vi "02_dosing.vi"() -> ()   [LabVIEW 2024]
uses:
  <vilib>/Utility/error.llb/DialogType.ctl
  <vilib>/Waveform/WDTOps.llb/WDT Waveform to XY Pairs DBL.vi
  <vilib>/Instr/_visa.llb/VISA Configure Serial Port (Instr).vi
  <vilib>/Utility/file.llb/Write Delimited Spreadsheet (string).vi
  <instrlib>/Tektronix DMM40x0 Series/Tektronix DMM40x0 Series.lvlib
panel:
  out "Waveform Graph":dbl[](graph)
  out "XY pairs":cluster{"x":timestamp, "y":dbl}[](array[cluster]) {"y" format="%0.2f"}
  in  "stop 2":bool
  in  "start   3":bool
  in  "pulse   2":bool
  in  "ready   2":bool
  in  "String 2":string
  out "String":string
  in  "Timeout (10000 ms)":u32=10000
  in  "Sample Count (10)":i32=10 format="%#.6g"
  in  "Trigger Count (5)":i32=5 format="%#.6g"
  in  "Function (0: DC Voltage)":u16(ring) items=["DC Voltage", "AC Voltage", "2 - Wire Resistance", "4 - Wire Resistance", "DC Current", "AC Current", "Frequency", "Period", "Continuity", "Diode Checking", "Temperature", "Capacitance"]
  in  "Serial Configuration":T1={"Baud Rate"=9600, "Parity"=0, "Data Bits"=8, "Stop Bits"=10, "Flow Control"=0} {"Flow Control" items=["None", "XON/XOFF", "RTS/CTS", "XON/XOFF & RTS/CTS", "DTR/DSR", "XON/XOFF & DTR/DSR"]; "Stop Bits" items=["1.0"=10, "1.5"=15, "2.0"=20]; "Data Bits" items=["7"=7, "8"=8]; "Parity" items=["None", "Odd", "Even", "Mark", "Space"]; "Baud Rate" items=["300"=300, "600"=600, "1200"=1200, "2400"=2400, "4800"=4800, "9600"=9600, "19200"=19200]}
  in  "VISA resource name":refnum<visa-resource-name>
  out "Data":string
  out "Array":string[](array[string])
  in  "SERIAL COMMAND":string(combo)
  out "PH METER OUTPUT":string
  in  "stop":bool
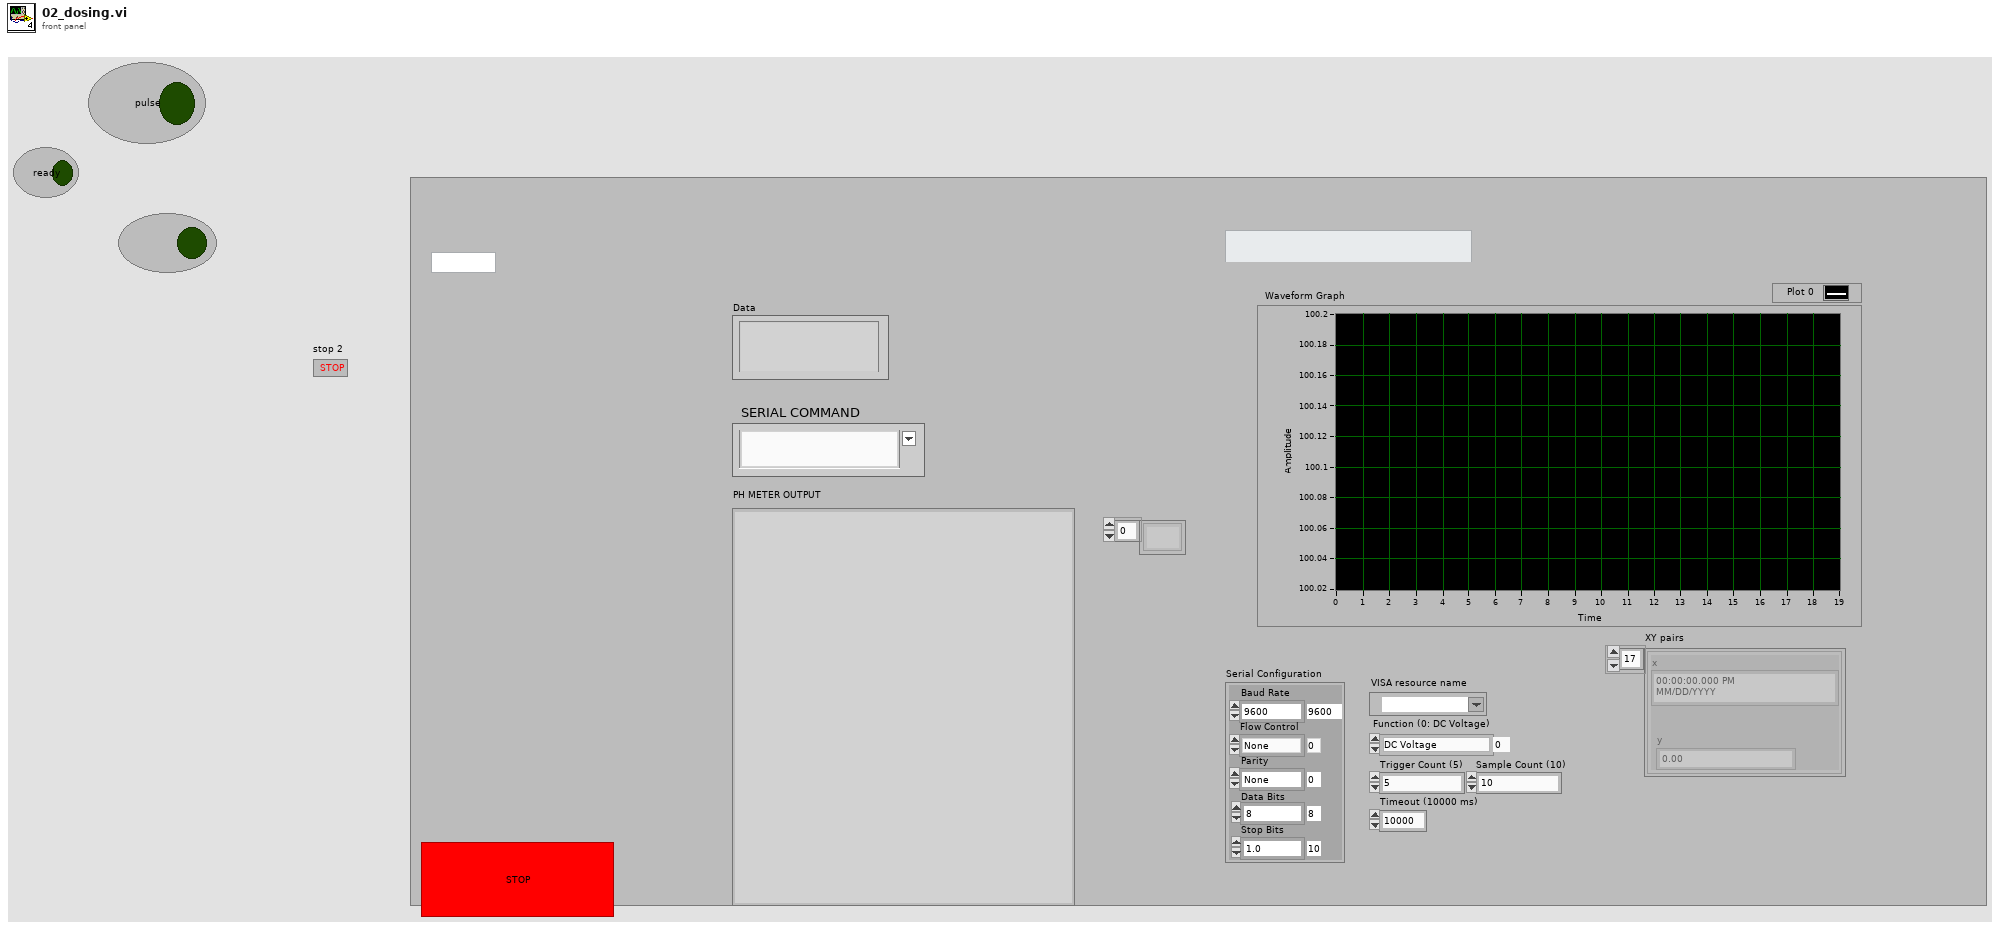
[diagram p1: front panel]
types:
  T1 = cluster{"Baud Rate":u32, "Parity":u16, "Data Bits":u16, "Stop Bits":u16, "Flow Control":u16}
  T2 = typedef "DialogType.ctl" = u16
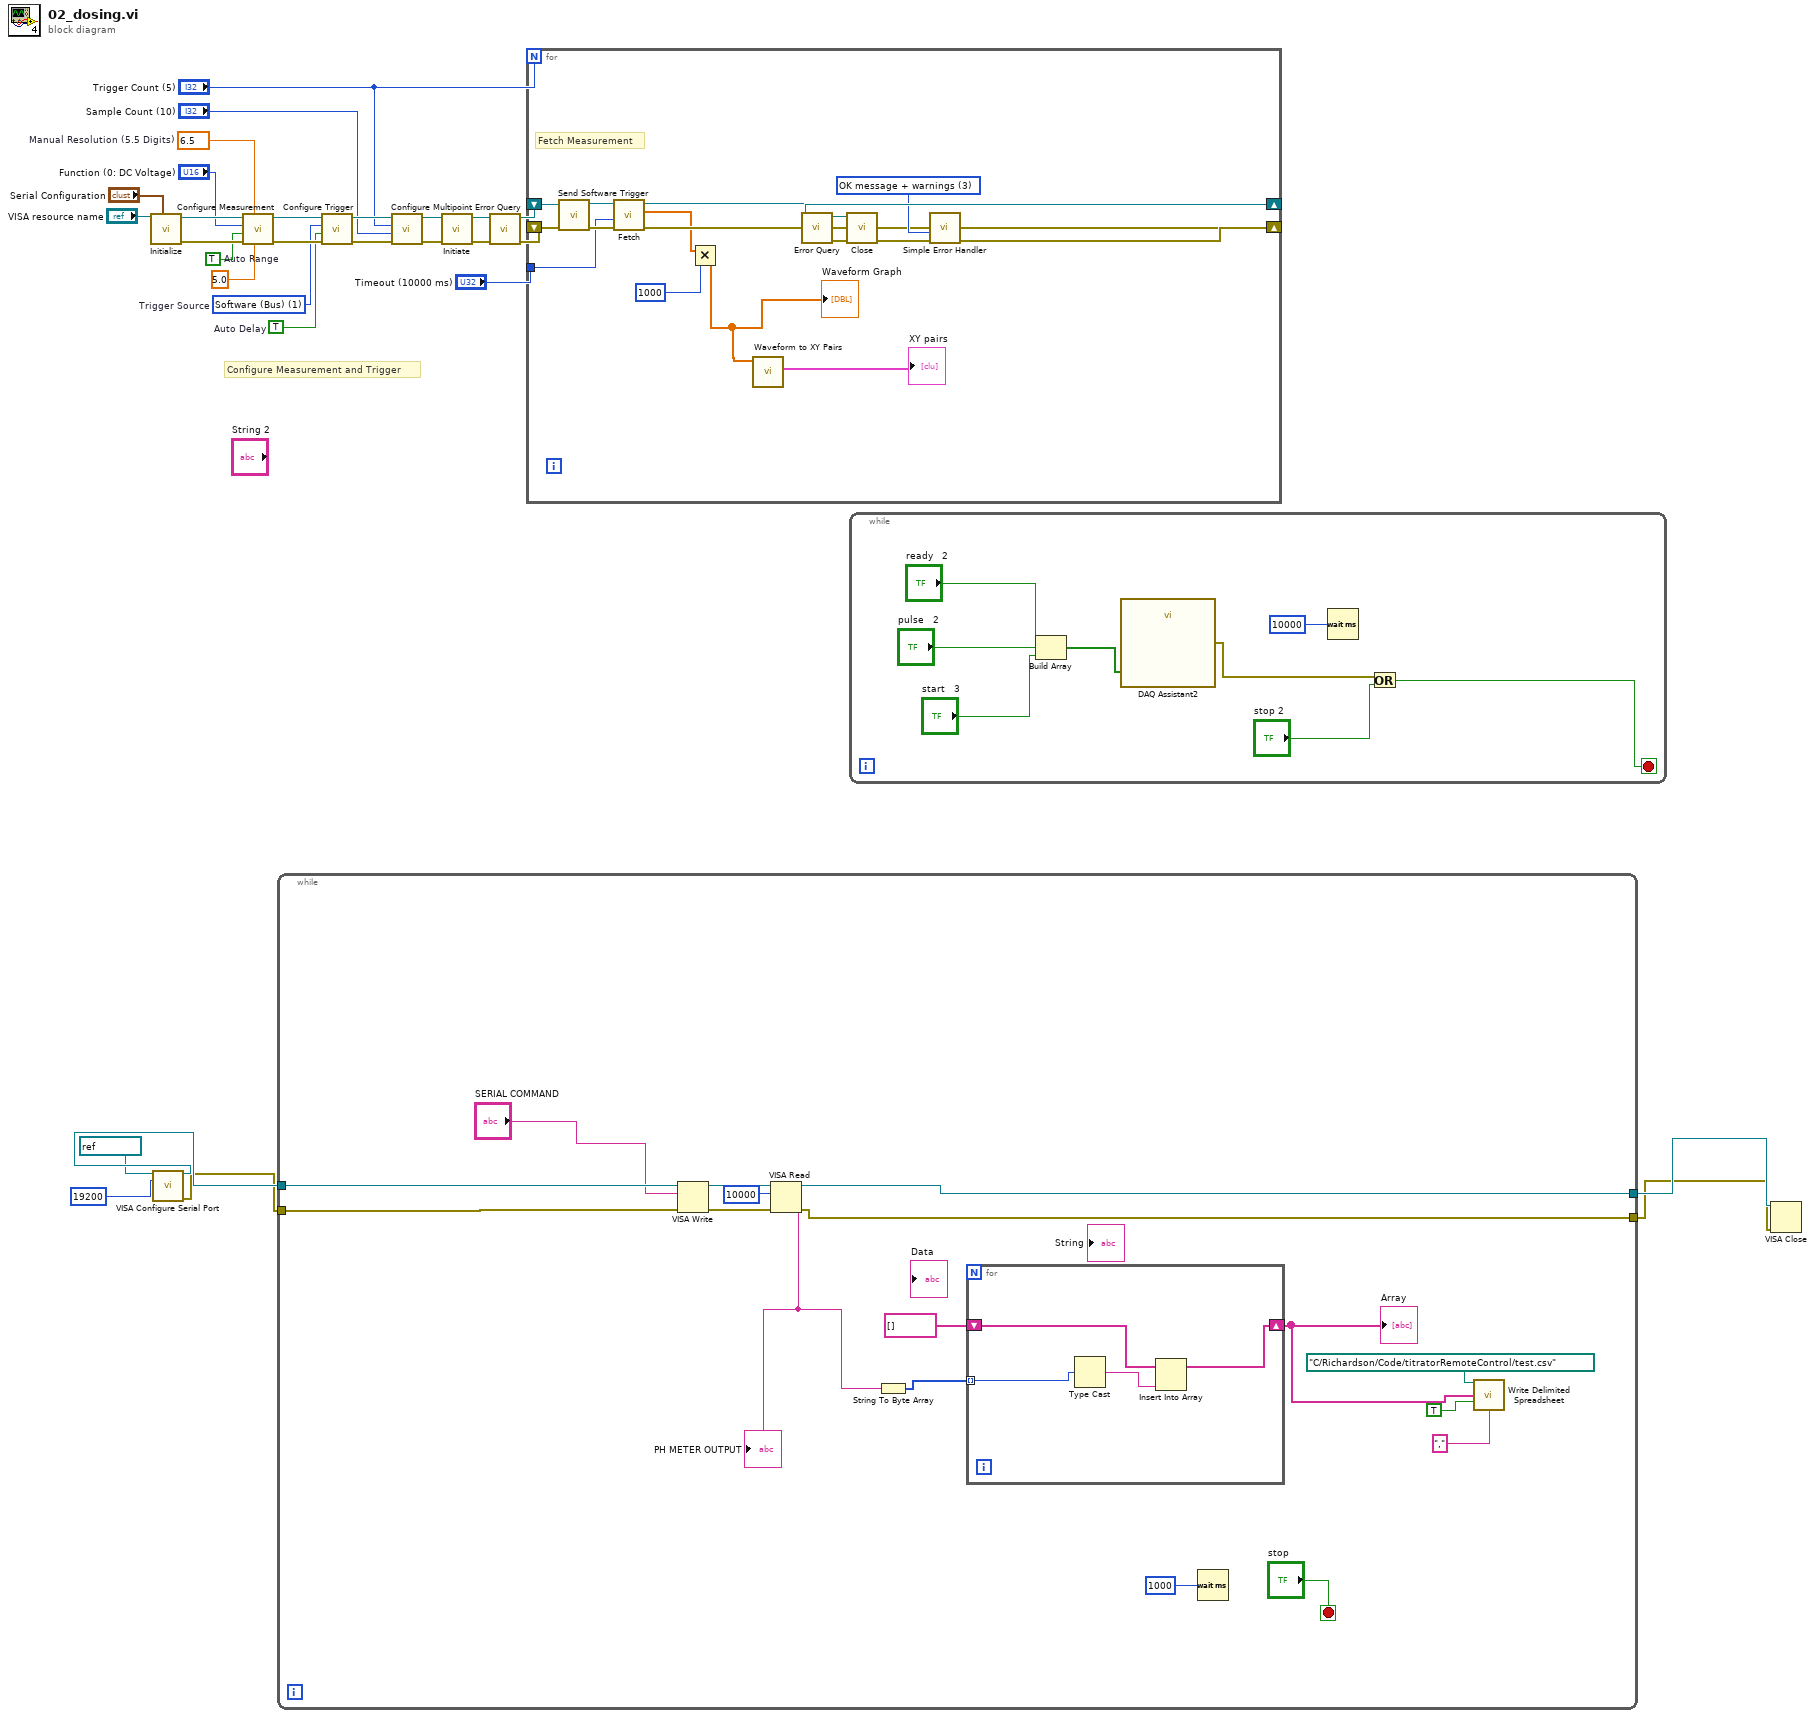
[diagram p0: block diagram]
diagram:
  w4 = 6.5 items=["4.5"=4.5, "5.5"=5.5, "6.5"=6.5]  # Manual Resolution (5.5 Digits)
  w12 = TRUE  # Auto Delay
  w13 = u16 1 items=["Immediate", "Software (Bus)", "External"]  # Trigger Source
  w14 = TRUE  # Auto Range
  w17 = T2 3 items=["no dialog", "OK message", "continue or stop message", "OK message + warnings", "continue/stop + warnings"] ("type of dialog (OK msg:1)")
  # "Configure Measurement and Trigger"
  n1 = call <instrlib>:"Initialize.vi"("Serial Configuration"="Serial Configuration", "VISA resource name"="VISA resource name") -> ("error out"=w29:errorcluster, "VISA resource name out"=w30:refnum<visa-resource-name>)  [unwired: 3 in, 5 out]
  n2 = call-poly "VISA Configure Serial Port"("VISA resource name"=refnum<visa-resource-name> "COM6", "baud rate (9600)"=u32 19200 ("byte count")) -> ("VISA resource name out"=w35:refnum<visa-resource-name>, "error out"=w33:errorcluster)  [unwired: 12 in]
  n3 = call <instrlib>:"Configure Measurement.vi"("Manual Range (1.0)"=5.0, "Manual Resolution (5.5 Digits)"=w4, "error in (no error)"=w29, "Auto Range (T:Enable)"=w14, "Function (0: DC Voltage)"="Function (0: DC Voltage)", "VISA resource name"=w30) -> ("error out"=w27:errorcluster, "VISA resource name out"=w28:refnum<visa-resource-name>)  [unwired: 4 out]
  n4 = while {
    tunnel: w35 -> [w50]
    tunnel: [w48] -> w34
    tunnel: w33 -> [w47]
    tunnel: [w45] -> w32
    stop <- "stop" stop-if-true
    n5 = VISA Write(VISA resource name=w50, write buffer="SERIAL COMMAND", error in (no error)=w47) -> (VISA resource name out=w49:refnum<visa-resource-name>, error out=w46:errorcluster)  [unwired: 1 out]
    n6 = VISA Read(VISA resource name=w49, byte count=u32 10000, error in (no error)=w46) -> (VISA resource name out=w48:refnum<visa-resource-name>, read buffer=w42:string, error out=w45:errorcluster)  [unwired: 1 out]
    "PH METER OUTPUT" <- w42
    n7 = String To Byte Array(string=w42) -> (unsigned byte array=w41:u8[])
    n8 = for {
      tunnel: w41 -> [w56] mode=indexing
      shift-right: [w53] -> w39
      shift-left: string[] [] -> [w55]
      n9 = Type Cast(x=w56) -> (*(type *) &x=w54:string)  [unwired: 1 in]
      n10 = Insert Into Array(array=w55, new element=w54) -> (w53:string[])  [unwired: 1 in]
    }
    "Array" <- w39
    n11 = Wait (ms)(milliseconds to wait=u32 1000 ("millisecond timer value")) -> ()  [unwired: 1 out]
    n12 = call-poly <vilib>:"Write Delimited Spreadsheet.vi"("file path (dialog if empty)"=path "C:/Richardson/Code/titratorRemoteControl/test.csv", "1D data"=w39, "append to file? (new file:F)"=TRUE, "delimiter (\\t)"="," ("delimiter (\\t)")) -> ()  [unwired: 10 in, 2 out]
  }
  n13 = call <instrlib>:"Configure Trigger.vi"("error in (no error)"=w27, "Auto Delay (T: Enable)"=w12, "Trigger Source (0: Immediate)"=w13, "VISA resource name"=w28) -> ("error out"=w25:errorcluster, "VISA resource name out"=w26:refnum<visa-resource-name>)  [unwired: 1 in, 5 out]
  n14 = call <instrlib>:"Configure Multipoint.vi"("error in (no error)"=w25, "Sample Count (1)"="Sample Count (10)", "Trigger Count (1)"="Trigger Count (5)", "VISA resource name"=w26) -> ("error out"=w22:errorcluster, "VISA resource name out"=w23:refnum<visa-resource-name>)  [unwired: 6 out]
  n15 = call <instrlib>:"Initiate.vi"("error in (no error)"=w22, "VISA resource name"=w23) -> ("error out"=w9:errorcluster, "VISA resource name out"=w8:refnum<visa-resource-name>)  [unwired: 8 out]
  n16 = call <instrlib>:"Error Query.vi"("error in (no error)"=w9, "VISA resource name"=w8) -> ("error out"=w6:errorcluster, "VISA resource name out"=w7:refnum<visa-resource-name>)  [unwired: 8 out]
  n17 = for {
    N: "Trigger Count (5)" -> [_]
    shift-right: [w66] -> w19
    shift-left: w6 -> [w62]
    shift-right: [w67] -> w21
    shift-left: w7 -> [w63]
    tunnel: "Timeout (10000 ms)" -> [w61]
    # "Fetch Measurement"
    n18 = call <instrlib>:"Send Software Trigger.vi"("error in (no error)"=w62, "VISA resource name"=w63) -> ("error out"=w64:errorcluster, "VISA resource name out"=w65:refnum<visa-resource-name>)  [unwired: 8 out]
    n19 = call <instrlib>:"Fetch.vi"("error in (no error)"=w64, "Timeout (10000 ms)"=w61, "VISA resource name"=w65) -> ("error out"=w66:errorcluster, "Measurements"=w60:dbl[], "VISA resource name out"=w67:refnum<visa-resource-name>)  [unwired: 6 out]
    n20 = Multiply(x=w60, y=1000) -> (x*y=w57:dbl[])
    "Waveform Graph" <- w57
    n21 = call-poly <vilib>:"Waveform to XY Pairs.vi"("waveform in"=w57) -> ("XY pairs"=→"XY pairs":cluster{"x":timestamp, "y":dbl}[])  [unwired: 8 in, 2 out]
  }
  n22 = call <instrlib>:"Error Query.vi"("error in (no error)"=w19, "VISA resource name"=w21) -> ("error out"=w18:errorcluster, "VISA resource name out"=w20:refnum<visa-resource-name>)  [unwired: 8 out]
  n23 = call <instrlib>:"Close.vi"("error in (no error)"=w18, "VISA resource name"=w20) -> ("error out"=w24:errorcluster)  [unwired: 9 out]
  n24 = while {
    stop <- w70 stop-if-true
    n25 = Build Array "Build Array"("ready   2", "pulse   2", "start   3") -> (w75:bool[])
    n26 = call "DAQ Assistant2"("data"=w75) -> ("error out"=w71:errorcluster)  [unwired: 17 in, 1 out]
    n27 = Wait (ms)(milliseconds to wait=u32 10000 ("millisecond timer value")) -> ()  [unwired: 1 out]
    n28 = Or(x=w71, y="stop 2") -> (x .or. y?=w70:bool)
  }
  n29 = call <vilib>:"Simple Error Handler.vi"("type of dialog (OK msg:1)"=w17, "error in (no error)"=w24) -> ()  [unwired: 8 out]
  n30 = VISA Close(VISA resource name=w34, error in (no error)=w32) -> ()  [unwired: 1 out]
